vi "CAN close.vi"(4 "error in (no error)":errorcluster, 7 "CANopen in":refnum<class "CANopen.lvclass">) -> (0 "error out":errorcluster)   [LabVIEW 2024]
doc: "Closes a previously established connection, freeing every allocated resouce. The closing step is executed independently of the error condition on input. The error out is a merge of the error in and the error returned by the close operation."
uses:
  CANopen.lvclass/CANopen.ctl
  CANopen.lvclass
panel:
  out "CANopen out":refnum<class "CANopen.lvclass">
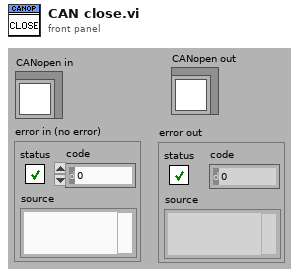
[diagram p1: front panel]
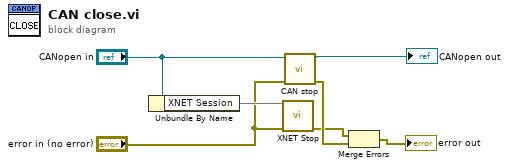
[diagram p0: block diagram]
diagram:
  n1 = Unbundle By Name("CANopen in") -> ("XNET Session"=w4)
  n2 = call <vilib>:"XNET Stop.vi"("session in"=w4, "error in (no error)"="error in (no error)") -> ("error out"=w1:errorcluster)  [unwired: 12 in, 1 out]
  n3 = call "CAN stop.vi"("error in (no error)"="error in (no error)", "CANopen in"="CANopen in") -> ("error out"=w7:errorcluster, "CANopen out"=→"CANopen out":refnum<class "CANopen.lvclass">)  [unwired: 4 out]
  n4 = Merge Errors(w1, w7) -> (→"error out":errorcluster)
